vi "Measurement Logic.vi"() -> ()   [LabVIEW 2024, in "NIScopeDigitalMeasurement.lvlib"]
uses:
  NIScopeDigitalMeasurement.lvlib
  Measurement Results.ctl
  <vilib>/MeasurementLink/MeasurementLink Measurement Server/Measure Call Context/Measure Call Context.lvclass
  Measurement Configuration.ctl
  <instrlib>/niScope/Controls/niScope scalar measurement.ctl
  <vilib>/MeasurementLink/MeasurementLink Measurement Server/Measure Call Context/Reserve Sessions - 1Pin.vi
  <vilib>/MeasurementLink/MeasurementLink niScope/Initialize Sessions - 1Sess.vi
  <vilib>/MeasurementLink/MeasurementLink niScope/Get Connections - 1Pin 1Conn.vi
  <instrlib>/niScope/Configure/Trigger/niScope Configure Trigger Edge.vi
  <instrlib>/niScope/Acquire/Fetch/niScope Fetch WDT.vi
  <vilib>/measure/mascope.llb/Amplitude and Levels 1 chan.vi
  <instrlib>/niScope/Measurements/niScope Fetch Measurement Stats.vi
  <vilib>/MeasurementLink/MeasurementLink niScope/MeasurementLink niScope.lvlib
  <vilib>/MeasurementLink/MeasurementLink Session Management V1/Session Reservation/Session Reservation.lvclass
  <vilib>/measure/NI_MAPro.lvlib
panel:
  in  "measurement configuration":T1={"Pin Name"="Pin1", "Vertical Range (V)"=10.0, "Vertical Offset (V)"=0.0, "Vertical Coupling"=1, "Minimum Sample Rate (S/s)"=1000000.0, "Minimum Record Length (S)"=2000, "Trigger Level (V)"=0.0, "Trigger Coupling"=0, "Trigger Slope"=1} {"Trigger Slope" items=["AC"=0, "DC"=1, "HF Reject"=3, "LF Reject"=4, "AC Plus HF Reject"=1001]; "Trigger Coupling" items=["Positive", "Negative"]; "Minimum Sample Rate (S/s)" format="%#.5p"; "Vertical Coupling" items=["AC", "DC", "Ground"]; "Vertical Offset (V)" format="%.2p"; "Vertical Range (V)" format="%.2f"}
  out "measure call context out":refnum<class "Measure Call Context.lvclass">
  in  "measure call context in":refnum<class "Measure Call Context.lvclass">
  out "measurement results":T2
  out "error out":errorcluster
  in  "error in":errorcluster
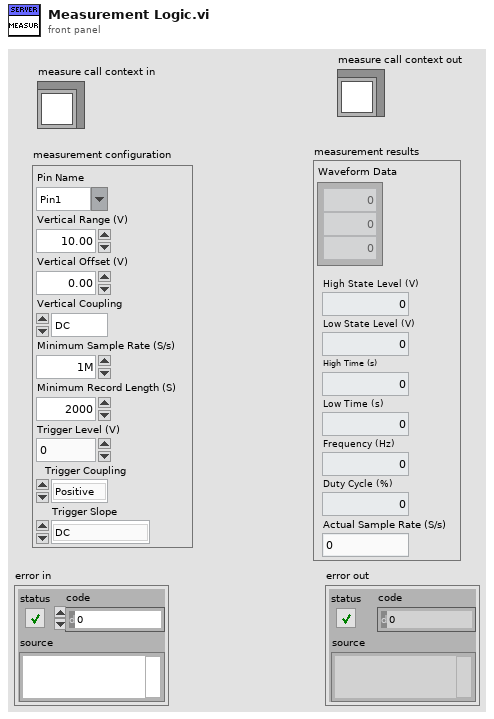
[diagram p1: front panel]
types:
  T1 = typedef "NIScopeDigitalMeasurement.lvlib/Measurement Configuration.ctl" = cluster{"Pin Name":string, "Vertical Range (V)":dbl, "Vertical Offset (V)":dbl, "Vertical Coupling":i32, "Minimum Sample Rate (S/s)":dbl, "Minimum Record Length (S)":i32, "Trigger Level (V)":dbl, "Trigger Coupling":u32, "Trigger Slope":i32}
  T2 = typedef "NIScopeDigitalMeasurement.lvlib/Measurement Results.ctl" = cluster{"Waveform Data":dbl[], "High Time (s)":dbl, "Low Time (s)":dbl, "Frequency (Hz)":dbl, "Duty Cycle (%)":dbl, "High State Level (V)":dbl, "Low State Level (V)":dbl, "Actual Sample Rate (S/s)":dbl}
  T3 = typedef "niScope scalar measurement.ctl" = i32
  T4 = typedef "MeasurementLink niScope.lvlib/Connection with Session.ctl" = cluster{"connection":T5, "session":refnum<k15>}
  T5 = typedef "MeasurementLink Session Management V1.lvlib/Session Reservation.lvclass/Connection.ctl" = cluster{"pin or relay name":string, "site":i32, "instrument type id":string, "channel":string}
  T6 = cluster{"result":dbl, "mean":dbl, "stdev":dbl, "min":dbl, "max":dbl, "num in stats":i32}
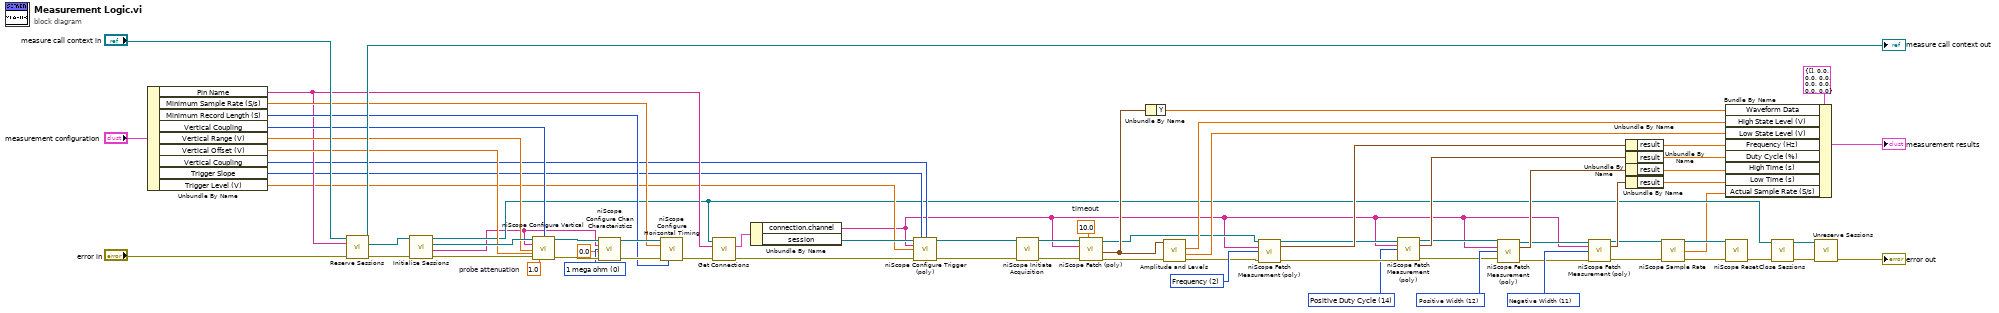
[diagram p0: block diagram]
diagram:
  w14 = T3 11 items=["None"=4000, "Frequency"=2, "Average Frequency"=1016, "FFT Frequency"=1008, "Period"=3, "Average Period"=1015, "Rise Time"=0, "Fall Time"=1, "Rising Slew Rate"=1010, "Falling Slew Rate"=1011, "Overshoot"=18, "Preshoot"=19, "Voltage RMS"=4, "Voltage Cycle RMS"=16, "AC Estimate"=1012, "FFT Amplitude"=1009, "Voltage Average"=10, "Voltage Cycle Average"=17, "DC Estimate"=1013, "Voltage Max"=6, "Voltage Min"=7, "Voltage Peak-to-Peak"=5, "Voltage High"=8, "Voltage Low"=9, "Voltage Amplitude"=15, "Voltage Top"=1007, "Voltage Base"=1006, "Voltage Base-to-Top"=1017, "Negative Width"=11, "Positive Width"=12, "Negative Duty Cycle"=13, "Positive Duty Cycle"=14, "Integral"=1005, "Area"=1003, "Cycle Area"=1004, "Time Delay"=1014, "Phase Delay"=1018, "Low Ref Volts"=1000, "Mid Ref Volts"=1001, "High Ref Volts"=1002, "Volt. Hist. Mean"=2000, "Volt. Hist. Stdev"=2001, "Volt. Hist. Median"=2003, "Volt. Hist. Mode"=2010, "Volt. Hist. Max"=2005, "Volt. Hist. Min"=2006, "Volt. Hist. Peak-to-Peak"=2002, "Volt. Hist. Mean + Stdev"=2007, "Volt. Hist. Mean + 2 Stdev"=2008, "Volt. Hist. Mean + 3 Stdev"=2009, "Volt. Hist. Hits"=2004, "Volt. Hist. New Hits"=2011, "Time Hist. Mean"=3000, "Time Hist. Stdev"=3001, "Time Hist. Median"=3003, "Time Hist. Mode"=3010, "Time Hist. Max"=3005, "Time Hist. Min"=3006, "Time Hist. Peak-to-Peak"=3002, "Time Hist. Mean + Stdev"=3007, "Time Hist. Mean + 2 Stdev"=3008, "Time Hist. Mean + 3 Stdev"=3009, "Time Hist. Hits"=3004, "Time Hist. New Hits"=3011] ("scalar measurement")
  w15 = T3 12 items=["None"=4000, "Frequency"=2, "Average Frequency"=1016, "FFT Frequency"=1008, "Period"=3, "Average Period"=1015, "Rise Time"=0, "Fall Time"=1, "Rising Slew Rate"=1010, "Falling Slew Rate"=1011, "Overshoot"=18, "Preshoot"=19, "Voltage RMS"=4, "Voltage Cycle RMS"=16, "AC Estimate"=1012, "FFT Amplitude"=1009, "Voltage Average"=10, "Voltage Cycle Average"=17, "DC Estimate"=1013, "Voltage Max"=6, "Voltage Min"=7, "Voltage Peak-to-Peak"=5, "Voltage High"=8, "Voltage Low"=9, "Voltage Amplitude"=15, "Voltage Top"=1007, "Voltage Base"=1006, "Voltage Base-to-Top"=1017, "Negative Width"=11, "Positive Width"=12, "Negative Duty Cycle"=13, "Positive Duty Cycle"=14, "Integral"=1005, "Area"=1003, "Cycle Area"=1004, "Time Delay"=1014, "Phase Delay"=1018, "Low Ref Volts"=1000, "Mid Ref Volts"=1001, "High Ref Volts"=1002, "Volt. Hist. Mean"=2000, "Volt. Hist. Stdev"=2001, "Volt. Hist. Median"=2003, "Volt. Hist. Mode"=2010, "Volt. Hist. Max"=2005, "Volt. Hist. Min"=2006, "Volt. Hist. Peak-to-Peak"=2002, "Volt. Hist. Mean + Stdev"=2007, "Volt. Hist. Mean + 2 Stdev"=2008, "Volt. Hist. Mean + 3 Stdev"=2009, "Volt. Hist. Hits"=2004, "Volt. Hist. New Hits"=2011, "Time Hist. Mean"=3000, "Time Hist. Stdev"=3001, "Time Hist. Median"=3003, "Time Hist. Mode"=3010, "Time Hist. Max"=3005, "Time Hist. Min"=3006, "Time Hist. Peak-to-Peak"=3002, "Time Hist. Mean + Stdev"=3007, "Time Hist. Mean + 2 Stdev"=3008, "Time Hist. Mean + 3 Stdev"=3009, "Time Hist. Hits"=3004, "Time Hist. New Hits"=3011] ("scalar measurement")
  w18 = T3 14 items=["None"=4000, "Frequency"=2, "Average Frequency"=1016, "FFT Frequency"=1008, "Period"=3, "Average Period"=1015, "Rise Time"=0, "Fall Time"=1, "Rising Slew Rate"=1010, "Falling Slew Rate"=1011, "Overshoot"=18, "Preshoot"=19, "Voltage RMS"=4, "Voltage Cycle RMS"=16, "AC Estimate"=1012, "FFT Amplitude"=1009, "Voltage Average"=10, "Voltage Cycle Average"=17, "DC Estimate"=1013, "Voltage Max"=6, "Voltage Min"=7, "Voltage Peak-to-Peak"=5, "Voltage High"=8, "Voltage Low"=9, "Voltage Amplitude"=15, "Voltage Top"=1007, "Voltage Base"=1006, "Voltage Base-to-Top"=1017, "Negative Width"=11, "Positive Width"=12, "Negative Duty Cycle"=13, "Positive Duty Cycle"=14, "Integral"=1005, "Area"=1003, "Cycle Area"=1004, "Time Delay"=1014, "Phase Delay"=1018, "Low Ref Volts"=1000, "Mid Ref Volts"=1001, "High Ref Volts"=1002, "Volt. Hist. Mean"=2000, "Volt. Hist. Stdev"=2001, "Volt. Hist. Median"=2003, "Volt. Hist. Mode"=2010, "Volt. Hist. Max"=2005, "Volt. Hist. Min"=2006, "Volt. Hist. Peak-to-Peak"=2002, "Volt. Hist. Mean + Stdev"=2007, "Volt. Hist. Mean + 2 Stdev"=2008, "Volt. Hist. Mean + 3 Stdev"=2009, "Volt. Hist. Hits"=2004, "Volt. Hist. New Hits"=2011, "Time Hist. Mean"=3000, "Time Hist. Stdev"=3001, "Time Hist. Median"=3003, "Time Hist. Mode"=3010, "Time Hist. Max"=3005, "Time Hist. Min"=3006, "Time Hist. Peak-to-Peak"=3002, "Time Hist. Mean + Stdev"=3007, "Time Hist. Mean + 2 Stdev"=3008, "Time Hist. Mean + 3 Stdev"=3009, "Time Hist. Hits"=3004, "Time Hist. New Hits"=3011] ("scalar measurement")
  w33 = T3 2 items=["None"=4000, "Frequency"=2, "Average Frequency"=1016, "FFT Frequency"=1008, "Period"=3, "Average Period"=1015, "Rise Time"=0, "Fall Time"=1, "Rising Slew Rate"=1010, "Falling Slew Rate"=1011, "Overshoot"=18, "Preshoot"=19, "Voltage RMS"=4, "Voltage Cycle RMS"=16, "AC Estimate"=1012, "FFT Amplitude"=1009, "Voltage Average"=10, "Voltage Cycle Average"=17, "DC Estimate"=1013, "Voltage Max"=6, "Voltage Min"=7, "Voltage Peak-to-Peak"=5, "Voltage High"=8, "Voltage Low"=9, "Voltage Amplitude"=15, "Voltage Top"=1007, "Voltage Base"=1006, "Voltage Base-to-Top"=1017, "Negative Width"=11, "Positive Width"=12, "Negative Duty Cycle"=13, "Positive Duty Cycle"=14, "Integral"=1005, "Area"=1003, "Cycle Area"=1004, "Time Delay"=1014, "Phase Delay"=1018, "Low Ref Volts"=1000, "Mid Ref Volts"=1001, "High Ref Volts"=1002, "Volt. Hist. Mean"=2000, "Volt. Hist. Stdev"=2001, "Volt. Hist. Median"=2003, "Volt. Hist. Mode"=2010, "Volt. Hist. Max"=2005, "Volt. Hist. Min"=2006, "Volt. Hist. Peak-to-Peak"=2002, "Volt. Hist. Mean + Stdev"=2007, "Volt. Hist. Mean + 2 Stdev"=2008, "Volt. Hist. Mean + 3 Stdev"=2009, "Volt. Hist. Hits"=2004, "Volt. Hist. New Hits"=2011, "Time Hist. Mean"=3000, "Time Hist. Stdev"=3001, "Time Hist. Median"=3003, "Time Hist. Mode"=3010, "Time Hist. Max"=3005, "Time Hist. Min"=3006, "Time Hist. Peak-to-Peak"=3002, "Time Hist. Mean + Stdev"=3007, "Time Hist. Mean + 2 Stdev"=3008, "Time Hist. Mean + 3 Stdev"=3009, "Time Hist. Hits"=3004, "Time Hist. New Hits"=3011] ("scalar measurement")
  w35 = 10.0  # timeout
  w63 = u32 0 items=["1 mega ohm"=0, "50 ohms"=2] ("input impedance")
  w66 = 1.0  # probe attenuation
  n1 = Unbundle By Name("measurement configuration") -> ("Pin Name"=w24:string, "Minimum Sample Rate (S/s)"=w47:dbl, "Minimum Record Length (S)"=w40:i32, "Vertical Coupling"=w48:i32, "Vertical Range (V)"=w49:dbl, "Vertical Offset (V)"=w50:dbl, "Vertical Coupling"=w21:i32, "Trigger Slope"=w20:i32, "Trigger Level (V)"=w19:dbl)
  n2 = call-poly <vilib>:"Reserve Sessions.vi"("error in"="error in", "pin or relay name"=w24, "measurement context in"="measure call context in") -> ("error out"=w70:errorcluster, "session reservation out"=w71:refnum<class "Session Reservation.lvclass">, "measurement context out"=→"measure call context out":refnum<class "Measure Call Context.lvclass">)  [unwired: 6 in]
  n3 = call-poly <vilib>:"Initialize Sessions.vi"("error in"=w70, "session reservation in"=w71) -> ("error out"=w67:errorcluster, "channel list"=w6:string, "session"=w60:refnum<k15>, "session reservation out"=w7:refnum<class "Session Reservation.lvclass">)  [unwired: 6 in]
  n4 = call <instrlib>:"niScope Configure Vertical.vi"("instrument handle"=w60, "probe attenuation"=w66, "vertical coupling"=w48, "channels"=w6, "vertical range"=w49, "vertical offset"=w50, "error in"=w67) -> ("instrument handle out"=w65:refnum<k15>, "error out"=w64:errorcluster)  [unwired: 7 in]
  n5 = call <instrlib>:"niScope Configure Chan Characteristics.vi"("instrument handle"=w65, "channels"=w6, "input impedance"=w63, "maximum input frequency"=0.0, "error in"=w64) -> ("instrument handle out"=w59:refnum<k15>, "error out"=w61:errorcluster)  [unwired: 9 in]
  n6 = call <instrlib>:"niScope Configure Horizontal Timing.vi"("instrument handle"=w59, "min sample rate"=w47, "error in"=w61, "min record length"=w40) -> ("error out"=w58:errorcluster)  [unwired: 10 in, 1 out]
  n7 = call-poly <vilib>:"Get Connections.vi"("error in"=w58, "pin or relay name"=w24, "session reservation in"=w7) -> ("error out"=w57:errorcluster, "connection"=w56:T4)  [unwired: 6 in, 1 out]
  n8 = Unbundle By Name(w56) -> ("connection.channel"=w8:string, "session"=w31:refnum<k15>)
  n9 = call-poly <instrlib>:"niScope Configure Trigger (poly).vi"("instrument handle"=w31, "trigger slope"=w20, "trigger coupling"=w21, "trigger source"=w8, "trigger level"=w19, "error in"=w57) -> ("instrument handle out"=w38:refnum<k15>, "error out"=w39:errorcluster)  [unwired: 8 in]
  n10 = call <instrlib>:"niScope Initiate Acquisition.vi"("instrument handle"=w38, "error in"=w39) -> ("instrument handle out"=w37:refnum<k15>, "error out"=w36:errorcluster)  [unwired: 12 in]
  n11 = call-poly <instrlib>:"niScope Fetch (poly).vi"("timeout"=w35, "error in"=w36, "channels"=w8, "instrument handle"=w37) -> ("error out"=w46:errorcluster, "wfm"=w45:waveform(dbl), "instrument handle out"=w32:refnum<k15>)  [unwired: 4 in, 1 out]
  n12 = Unbundle By Name(w45) -> ("Y"=w44:dbl[])
  n13 = call-poly <vilib>:"Amplitude and Levels.vi"("error in (no error)"=w46, "signal in"=w45) -> ("error out"=w29:errorcluster, "low state level"=w42:dbl, "high state level"=w43:dbl)  [unwired: 6 in, 1 out]
  n14 = call-poly <instrlib>:"niScope Fetch Measurement (poly).vi"("instrument handle"=w32, "channels"=w8, "scalar measurement"=w33, "error in"=w29) -> ("instrument handle out"=w30:refnum<k15>, "stats"=w34:T6, "error out"=w23:errorcluster)  [unwired: 9 in]
  n15 = call-poly <instrlib>:"niScope Fetch Measurement (poly).vi"("instrument handle"=w30, "channels"=w8, "scalar measurement"=w18, "error in"=w23) -> ("instrument handle out"=w11:refnum<k15>, "stats"=w17:T6, "error out"=w12:errorcluster)  [unwired: 9 in]
  n16 = call-poly <instrlib>:"niScope Fetch Measurement (poly).vi"("instrument handle"=w11, "channels"=w8, "scalar measurement"=w15, "error in"=w12) -> ("instrument handle out"=w10:refnum<k15>, "stats"=w16:T6, "error out"=w9:errorcluster)  [unwired: 9 in]
  n17 = call-poly <instrlib>:"niScope Fetch Measurement (poly).vi"("instrument handle"=w10, "channels"=w8, "scalar measurement"=w14, "error in"=w9) -> ("instrument handle out"=w3:refnum<k15>, "stats"=w13:T6, "error out"=w4:errorcluster)  [unwired: 9 in]
  n18 = Unbundle By Name(w34) -> ("result"=w28:dbl)
  n19 = Unbundle By Name(w17) -> ("result"=w27:dbl)
  n20 = Unbundle By Name(w16) -> ("result"=w26:dbl)
  n21 = Unbundle By Name(w13) -> ("result"=w25:dbl)
  n22 = call <instrlib>:"niScope Sample Rate.vi"("instrument handle"=w3, "error in"=w4) -> ("instrument handle out"=w2:refnum<k15>, "actual sample rate"=w1:dbl, "error out"=w5:errorcluster)  [unwired: 11 in]
  n23 = call <instrlib>:"niScope Reset.vi"("instrument handle"=w2, "error in"=w5) -> ("error out"=w55:errorcluster)  [unwired: 12 in, 1 out]
  n24 = Bundle By Name(cluster=T2 {"Waveform Data"=[], "High Time (s)"=0.0, "Low Time (s)"=0.0, "Frequency (Hz)"=0.0, "Duty Cycle (%)"=0.0, "High State Level (V)"=0.0, "Low State Level (V)"=0.0, "Actual Sample Rate (S/s)"=0.0} ("measurement results"), "Waveform Data"=w44, "High State Level (V)"=w43, "Low State Level (V)"=w42, "Frequency (Hz)"=w28, "Duty Cycle (%)"=w27, "High Time (s)"=w26, "Low Time (s)"=w25, "Actual Sample Rate (S/s)"=w1) -> (→"measurement results":T2)
  n25 = call <vilib>:"Close Sessions.vi"("error in"=w55, "session reservation in"=w7) -> ("error out"=w68:errorcluster, "session reservation out"=w69:refnum<class "Session Reservation.lvclass">)  [unwired: 8 in]
  n26 = call <vilib>:"Unreserve Sessions.vi"("error in"=w68, "session reservation in"=w69) -> ("error out"=→"error out":errorcluster)  [unwired: 9 in]
